vi "zad3 - v0.0.1.vi"() -> ()   [LabVIEW 2017]
panel:
  in  "Prąd [A]":dbl min=0.0 max=0.00113
  in  "TRYB":i16(knob) step=1 scale=1.0..2.0
  in  "DAC0":dbl(knob) scale=0.04..2.5
  out "Rs":dbl
  in  "Interval (ms)":u32=500
  in  "stop":bool
  out "AIN3":dbl format="%.6f"
  out "AIN2":dbl format="%.6f"
  in  "FIO7":bool
  in  "FIO6":bool
  out "Error Message":string
  out "error out":errorcluster
  # "Outputs DAC0 and FIO6-FIO7.  Aquires AIN0-AIN3 and FIO4-FIO5.  This example\ndoes the proper pin configuration also.  Uses USB on the first found U3."
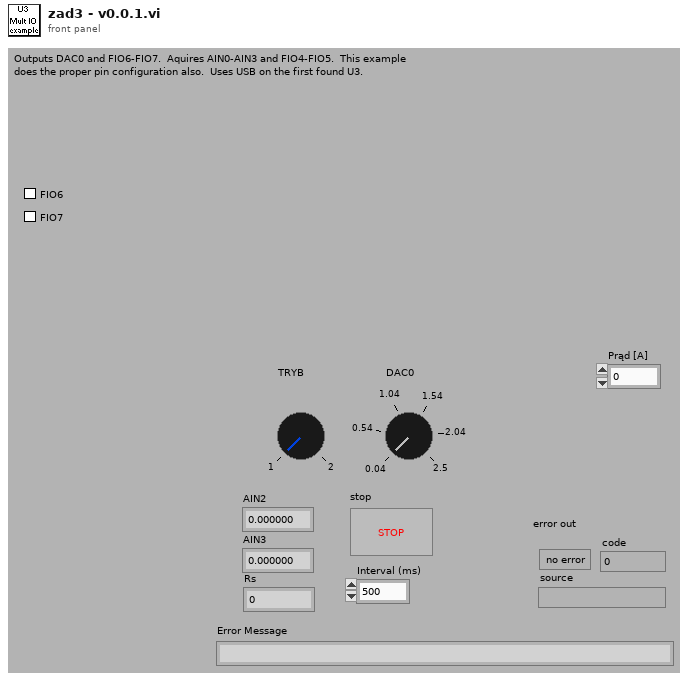
[diagram p1: front panel]
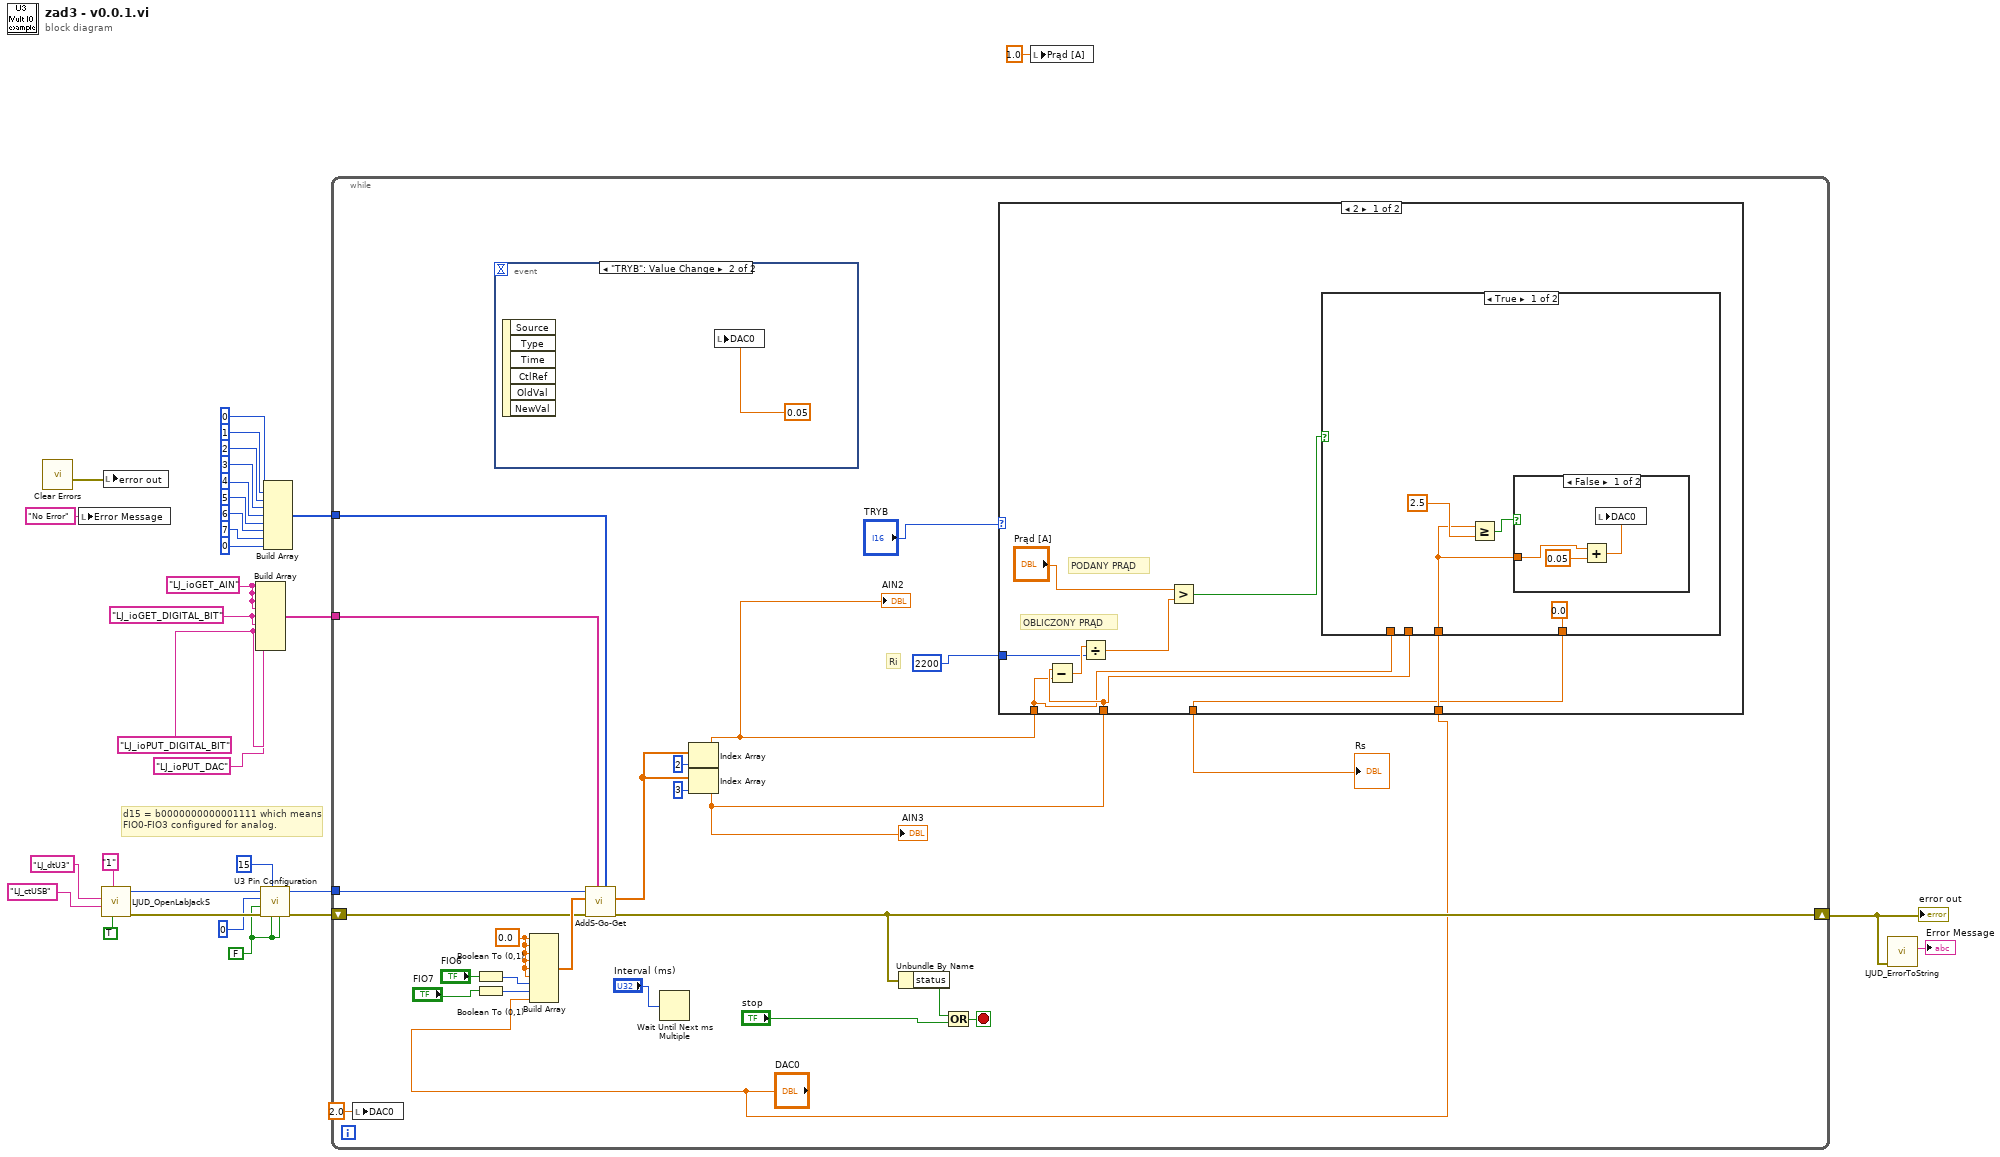
[diagram p0: block diagram]
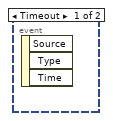
[diagram p2: hidden frame]
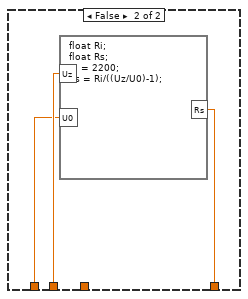
[diagram p4: hidden frame]
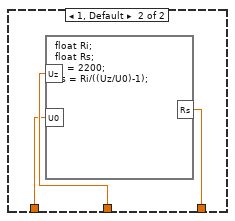
[diagram p5: hidden frame]
diagram:
  w5 = FALSE ("Enable DAC1")
  w29 = "LJ_ioPUT_DIGITAL_BIT" ("IOType")
  w31 = "LJ_ioGET_AIN" ("IOType")
  w30 = "LJ_ioGET_DIGITAL_BIT" ("IOType")
  # "d15 = b0000000000001111 which means\nFIO0-FIO3 configured for analog."
  n1 = call <vilib>:"Clear Errors.vi"() -> ("error out"=w3:errorcluster)  [unwired: 6 in, 1 out]
  n2 = local write "Error Message"("No Error" ("Error Message")) -> ()
  n3 = call "LJUD_OpenLabJackS.vi"("FirstFound"=TRUE, "Address"="1", "ConnectionType"="LJ_ctUSB", "DeviceType"="LJ_dtU3") -> ("error out"=w10:errorcluster, "Handle"=w8:i32)  [unwired: 5 in, 1 out]
  n4 = local write "error out"(w3) -> ()
  n5 = Build Array(w31, w31, w31, w31, w30, w30, w29, w29, "LJ_ioPUT_DAC" ("IOType")) -> (w28:string[])
  n6 = call "U3 Pin Configuration.vi"("Enable Counter1"=w5, "Enable Counter0"=w5, "FIO/EIO Analog Enable"=15, "error in"=w10, "Enable DAC1"=w5, "Number of Timers Enabled"=u8 0, "Handle In"=w8) -> ("error out"=w11:errorcluster, "Handle Out"=w9:i32)  [unwired: 3 in]
  n7 = Build Array(0, 1, 2, 3, 4, 5, 6, 7, 0) -> (w27:i32[])
  n8 = while {
    shift-left: w11 -> [w41]
    shift-right: [w40] -> w12
    tunnel: w9 -> [w45]
    tunnel: w27 -> [w55]
    tunnel: w28 -> [w56]
    stop <- w44 stop-if-true
    w54 = 0.0 ("Input Element")
    # "Ri"
    n9 = Boolean To (0,1)(Boolean="FIO6") -> (0, 1=w53:i16)
    n10 = Boolean To (0,1)(Boolean="FIO7") -> (0, 1=w52:i16)
    n11 = event shown="[1] \"TRYB\": Value Change" {
      selector: _ -> [_ _]
      dyn-events: _ -> [_ _]
      timeout: _ -> [_ _]
      event Timeout {
        n12 = event-data() -> ()  [unwired: 1 in, 3 out]
      }
      event "TRYB": Value Change {
        n13 = event-data() -> ()  [unwired: 1 in, 6 out]
        n14 = local write "DAC0"(0.05 ("DAC0")) -> ()
      }
    }
    n15 = Build Array(w54, w54, w54, w54, w54, w54, w53, w52, "DAC0") -> (w51:dbl[])
    n16 = call "AddS-Go-Get.vi"("Channels"=w55, "IOTypes"=w56, "error in"=w41, "Values Write"=w51, "Handle In"=w45) -> ("error out"=w40:errorcluster, "Values Read"=w48:dbl[])  [unwired: 4 in, 1 out]
    n17 = Wait Until Next ms Multiple(millisecond multiple="Interval (ms)") -> ()  [unwired: 1 out]
    n18 = Index Array(array=w48, index=2 ("Index")) -> (element=w37:dbl)
    "AIN2" <- w37
    n19 = Index Array(array=w48, index=3 ("Index")) -> (element=w38:dbl)
    "AIN3" <- w38
    n20 = Unbundle By Name(w40) -> ("status"=w42:bool)
    n21 = Or(x=w42, y="stop") -> (x .or. y?=w44:bool)
    n22 = case shown="2" "TRYB" {
      tunnel: w38 -> [w60 w79]
      tunnel: w37 -> [w59 w78]
      tunnel: [w58 w77] -> w36
      tunnel: 2200 -> [w65 _]
      tunnel: "DAC0" -> [w61 _]
      frame 2 {
        # "PODANY PRĄD"
        # "OBLICZONY PRĄD"
        n23 = Subtract(x=w60, y=w59) -> (x-y=w66:dbl)
        n24 = Divide(x=w66, y=w65) -> (x/y=w63:dbl)
        n25 = Greater?(x="Prąd [A]", y=w63) -> (0:w62:bool)
        n26 = case shown="True" w62 {
          tunnel: w61 -> [w68 _]
          tunnel: w60 -> [_ w76]
          tunnel: w59 -> [_ w75]
          tunnel: [0.0 w74] -> w58
          frame True {
            n27 = Greater Or Equal?(x=w68, y=2.5) -> (x >= y?=w69:bool)
            n28 = case shown="False" w69 {
              tunnel: w68 -> [w71 _]
              frame False {
                n29 = Add(x=w71, y=0.05) -> (x+y=w73:dbl)
                n30 = local write "DAC0"(w73) -> ()
              }
              frame True {
              }
            }
          }
          frame False {
            n31 = formula code="float Ri;\nfloat Rs;\nRi = 2200;\nRs = Ri/((Uz/U0)-1);"("Uz"=w76, "U0"=w75) -> ("Rs"=w74:dbl)
          }
        }
      }
      frame 1, Default {
        n32 = formula code="float Ri;\nfloat Rs;\nRi = 2200;\nRs = Ri/((Uz/U0)-1);"("Uz"=w79, "U0"=w78) -> ("Rs"=w77:dbl)
      }
    }
    "Rs" <- w36
  }
  "error out" <- w12
  n33 = local write "DAC0"(2.0 ("DAC0")) -> ()
  n34 = local write "Prąd [A]"(1.0 ("Prąd [A]")) -> ()
  n35 = call "LJUD_ErrorToString.vi"("error in"=w12) -> ("String"=→"Error Message":string)  [unwired: 10 in]
